vi "Bundle Data Log.vi"(0 "DSA Measurements":T7[][](array[typedef]), 1 "WT1800 Measurements":T4[][](array[typedef]) {"Vrms" format="%.3f"; "Irms" format="%.3f"; "Power" format="%.3f"; "Vpkpk" format="%.3f"; "Ipkpk" format="%.3f"}, 2 "DSA Averages":T6, 3 "WT1800 Averages":T3 {"Vrms" format="%.3f"; "Irms" format="%.3f"; "Power" format="%.3f"; "Vpkpk" format="%.3f"; "Ipkpk" format="%.3f"}, 5 "WT1800 Functions":T2, 7 "DSA Functions":T5, 9 "Temperature Data":dbl[][](array[numeric]), 11 "error in (no error)":errorcluster, 12 "Error or Abort":bool, 13 "Run Mode (Manual = True)":bool) -> (4 "Average Power + Heat":dbl[](array[numeric]) format="%.3g", 6 "Heat":dbl, 10 "Datalog Cluster":T1 {"WT1800 Averages"."Vrms" format="%.3f"; "WT1800 Averages"."Irms" format="%.3f"; "WT1800 Averages"."Power" format="%.3f"; "WT1800 Averages"."Vpkpk" format="%.3f"; "WT1800 Averages"."Ipkpk" format="%.3f"; "WT1800 Measurements"."Vrms" format="%.3f"; "WT1800 Measurements"."Irms" format="%.3f"; "WT1800 Measurements"."Power" format="%.3f"; "WT1800 Measurements"."Vpkpk" format="%.3f"; "WT1800 Measurements"."Ipkpk" format="%.3f"; "DSA Averages"."Vrms" format="%.3f"; "DSA Averages"."Vdc" format="%.3f"; "DSA Averages"."Vpk+" format="%.3f"; "DSA Averages"."Vpk-" format="%.3f"; "DSA Averages"."Vpkpk" format="%.3f"; "DSA Measurements"."Vrms" format="%.3f"; "DSA Measurements"."Vdc" format="%.3f"; "DSA Measurements"."Vpk+" format="%.3f"; "DSA Measurements"."Vpk-" format="%.3f"; "DSA Measurements"."Vpkpk" format="%.3f"}, 14 "Error or Abort Out":bool, 15 "error out":errorcluster)   [LabVIEW 2021]
uses:
  Controls/WT1800 Readings.ctl
  Controls/WT1800 Measurements.ctl
  Controls/WT1800 Functions.ctl
  Controls/DSA Measurements.ctl
  Controls/DSA Readings.ctl
  Controls/DSA Functions.ctl
  Controls/Datalog Bundle Control.ctl
panel:
  in  "Initial Time Stamp":timestamp
  in  "Final Time Stamp":timestamp
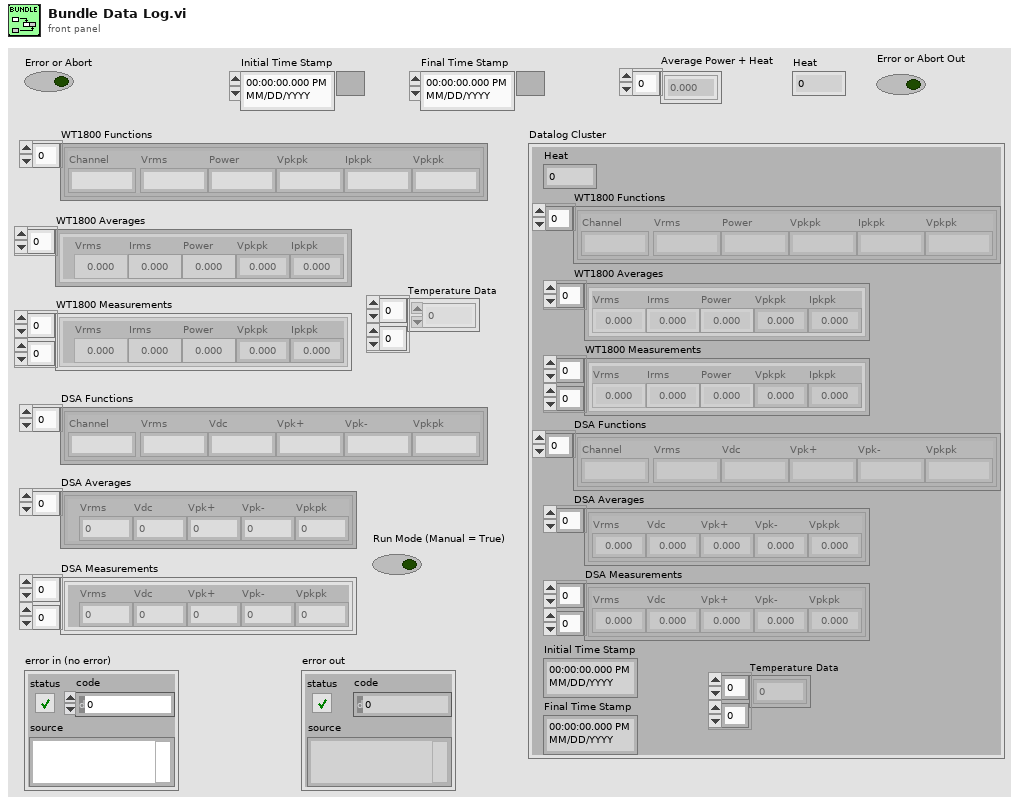
[diagram p1: front panel]
types:
  T1 = typedef "Datalog Bundle Control.ctl" = cluster{"Heat":dbl, "WT1800 Functions":T2, "WT1800 Averages":T3, "WT1800 Measurements":T4[][], "DSA Functions":T5, "DSA Averages":T6, "DSA Measurements":T7[][], "Initial Time Stamp":timestamp, "Final Time Stamp":timestamp, "Temperature Data":sgl[][]}
  T2 = typedef "WT1800 Functions.ctl" = cluster{"Channel":string, "Vrms":string, "Power":string, "Vpkpk":string, "Ipkpk":string, "Vpkpk":string}[]
  T3 = typedef "WT1800 Measurements.ctl" = T4[]
  T4 = typedef "WT1800 Readings.ctl" = cluster{"Vrms":sgl, "Irms":sgl, "Power":sgl, "Vpkpk":sgl, "Ipkpk":sgl}
  T5 = typedef "DSA Functions.ctl" = cluster{"Channel":string, "Vrms":string, "Vdc":string, "Vpk+":string, "Vpk-":string, "Vpkpk":string}[]
  T6 = typedef "DSA Measurements.ctl" = T7[]
  T7 = typedef "DSA Readings.ctl" = cluster{"Vrms":sgl, "Vdc":sgl, "Vpk+":sgl, "Vpk-":sgl, "Vpkpk":sgl}
  T8 = cluster{dbl, "WT1800 Functions":T2, "WT1800 Averages":T3, "WT1800 Measurements":T4[][], "DSA Functions":T5, "DSA Averages":T6, "DSA Measurements":T7[][], "Initial Time Stamp":timestamp, "Final Time Stamp":timestamp, "Temperature Data":dbl[][]}
  T9 = cluster{sgl, "WT1800 Functions":T2, "WT1800 Averages":T3, "WT1800 Measurements":T4[][], "DSA Functions":T5, "DSA Averages":T6, "DSA Measurements":T7[][], "Initial Time Stamp":timestamp, "Final Time Stamp":timestamp, "Temperature Data":dbl[][]}
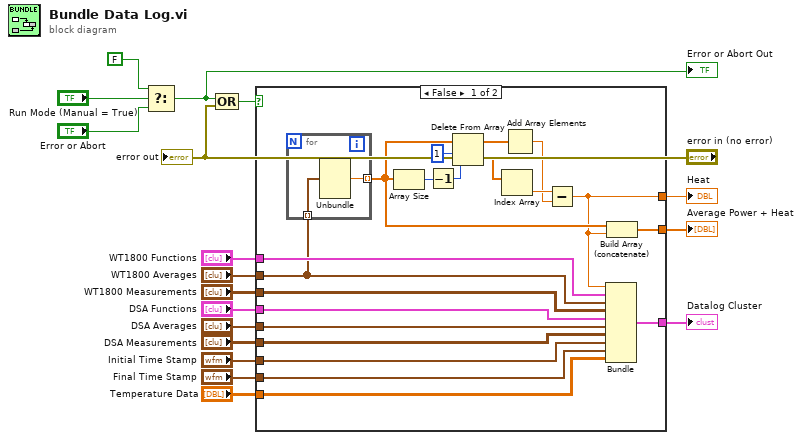
[diagram p0: block diagram]
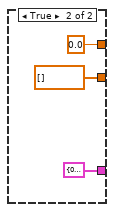
[diagram p2: hidden frame]
diagram:
  n1 = Select(t=FALSE, s="Run Mode (Manual = True)", f="Error or Abort") -> (s? t:f=w1:bool)
  "Error or Abort Out" <- w1
  n2 = Compound Arithmetic op=OR(w1, "error in (no error)") -> (w7:bool)
  n3 = case shown="False" w7 {
    tunnel: "WT1800 Measurements" -> [w27 _]
    tunnel: "WT1800 Functions" -> [w38 _]
    tunnel: "Initial Time Stamp" -> [w22 _]
    tunnel: "Final Time Stamp" -> [w37 _]
    tunnel: "DSA Functions" -> [w25 _]
    tunnel: "DSA Measurements" -> [w24 _]
    tunnel: "DSA Averages" -> [w26 _]
    tunnel: "WT1800 Averages" -> [w28 _]
    tunnel: [w23 dbl[] []] -> w10
    tunnel: [w21 0.0] -> w9
    tunnel: [w20 T8 {0.0, "WT1800 Functions"=[], "WT1800 Averages"=[], "WT1800 Measurements"=[], "DSA Functions"=[], "DSA Averages"=[], "DSA Measurements"=[], "Initial Time Stamp"=timestamp(0 s since 1904-01-01), "Final Time Stamp"=timestamp(0 s since 1904-01-01), "Temperature Data"=[]}] -> w8
    tunnel: "Temperature Data" -> [w19 _]
    frame False {
      n4 = for {
        tunnel: w28 -> [w40] mode=indexing
        tunnel: [w39] -> w35 mode=indexing
        n5 = Unbundle(w40) -> ("Power"=w39:sgl)  [unwired: 4 out]
      }
      n6 = Array Size(array=w35) -> (size(s)=w33:i32)
      n7 = Decrement(x=w33) -> (x-1=w32:i32)
      n8 = Delete From Array(array=w35, length=1, index=w32) -> (deleted portion=w31:sgl[], array with subset deleted=w34:sgl[])
      n9 = Index Array(array=w31) -> (element=w30:sgl)  [unwired: 1 in]
      n10 = Add Array Elements(numeric array=w34) -> (sum=w29:sgl)
      n11 = Subtract(x=w30, y=w29) -> (x-y=w21:sgl)
      n12 = Bundle(w21, "WT1800 Functions"=w38, "WT1800 Averages"=w28, "WT1800 Measurements"=w27, "DSA Functions"=w25, "DSA Averages"=w26, "DSA Measurements"=w24, "Initial Time Stamp"=w22, "Final Time Stamp"=w37, "Temperature Data"=w19) -> (w20:T9)  [unwired: 1 in]
      n13 = Build Array (concatenate)(w35, w21) -> (w23:sgl[])
    }
    frame True {
    }
  }
  "Average Power + Heat" <- w10
  "Heat" <- w9
  "Datalog Cluster" <- w8
  "error out" <- "error in (no error)"
